vi "Build Configuration Error String.vi"(7 "Name":string, 8 "error in (no error)":errorcluster, 9 "String in":string, 10 "Error":string, 11 "Error?":bool) -> (0 "error out":errorcluster, 1 "String out":string)   [LabVIEW 2019, in "Diagnostics Addon System Explorer.lvlib"]
uses:
  Diagnostics Addon System Explorer.lvlib
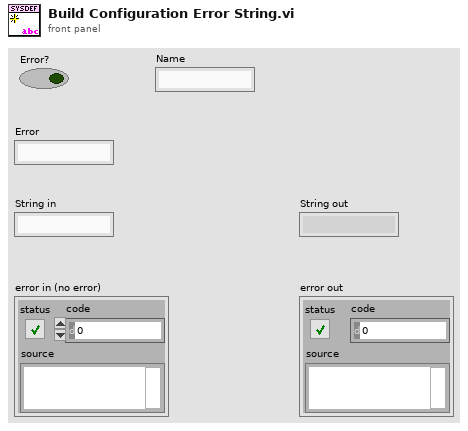
[diagram p1: front panel]
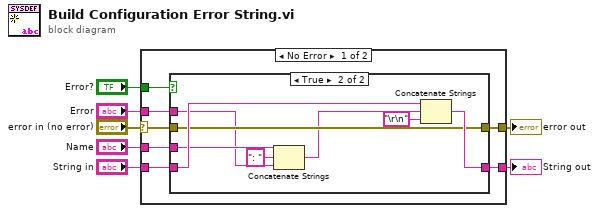
[diagram p0: block diagram]
diagram:
  n1 = case shown="No Error" "error in (no error)" {
    selector: "error in (no error)" -> [w10 w25]
    tunnel: "Error?" -> [w13 _]
    tunnel: "Error" -> [w14 _]
    tunnel: [w12 w26] -> w1
    tunnel: "String in" -> [w11 w26]
    tunnel: [w9 w25] -> w3
    tunnel: "Name" -> [w8 _]
    frame No Error {
      n2 = case shown="True" w13 {
        tunnel: w14 -> [_ w18]
        tunnel: [w16 w24] -> w12
        tunnel: w11 -> [w16 w23]
        tunnel: w10 -> [w15 w21]
        tunnel: [w15 w21] -> w9
        tunnel: w8 -> [_ w20]
        frame False {
        }
        frame True {
          n3 = Concatenate Strings(w20, ": " ("string"), w18) -> (w17:string)
          n4 = Concatenate Strings(w23, w17, "\r\n") -> (w24:string)
        }
      }
    }
    frame Error {
    }
  }
  "error out" <- w3
  "String out" <- w1
